vi "Rx Async.vi"(8 "error in (no error)":errorcluster, 11 "Framework in":refnum<class "Framework.lvclass">) -> (0 "error out":errorcluster, 3 "Framework out":refnum<class "Framework.lvclass">)   [LabVIEW 2017, in "DSF Core.lvlib" / "Framework.lvclass"]
uses:
  Framework.lvclass
  Framework.lvclass/Framework.ctl
  Plugin/Plugin.lvclass/Plugin.ctl
  Transfer Group/Transfer Group.lvclass/Transfer Group.ctl
  Timing/Timing.lvclass/Timing.ctl
  Buffers/Buffers.lvclass/Buffers.ctl
  Interfaces/Interface/Interface.lvclass/Interface.ctl
  Transfer Group/Increment Iteration.vi
  Transfer Group/Get Iteration.vi
  Dispatcher/Dispatch Transfer Group.vi
  Transfer Group/Get ID.vi
  Transfer Group/Copy Async to Inline.vi
  Transfer Group/Wait For Previous.vi
  Transfer Group/Update Status.vi
  Transfer Group/Get Active.vi
  Timing/Increment Iteration.vi
  Timing/Get Iteration.vi
  Interfaces/Dispatcher/Send Dispatcher Command.vi
  Buffers/Copy Async to Inline.vi
  Transfer Group/Retrieve from FIFO.vi
  Transfer Group Status/Write Status.vi
  Interfaces/Dispatcher/Write.vi
  Interfaces/Dispatcher/Write Dispatcher Command.vi
  Transfer Group/Read Return FIFO.vi
  Transfer Group/Increment Late Count.vi
  Transfer Group Status/Status Size.vi
  Interfaces/Interface/Send Command.vi
  Interfaces/Interface/Write RT FIFO.vi
  Buffer/Buffer.lvclass
  C:/Git/DSF/LabVIEW-Memory/Source/Classes/Pointer/Pointer.lvclass
  Interfaces/Dispatcher/Dispatcher Interface.lvclass
  C:/Git/DSF/Data Sharing Framework Core/Classes/Interfaces/Interface/Interface.lvclass
  Transfer Group Status/Status.lvclass
  LabVIEW-Memory/Source/Classes/Pointer/Get Address.vi
  LabVIEW-Memory/Source/Classes/Pointer/Check Size (0D).vi
  LabVIEW-Memory/Source/Classes/Pointer/Check Null Pointer.vi
  Interfaces/Interface/Errors.vi
  Interfaces/Dispatcher/Command Timeout.vi
  VIs/VI Name.vi
  Interfaces/Dispatcher/Class Name.vi
  LabVIEW-Memory/Source/Classes/Pointer/Copy All.vi
  Transfer Group/Errors.vi
  Transfer Group/Return Timeout Error.vi
  Transfer Group/Invalid Iteration Error.vi
  Plugin/Plugin.lvclass
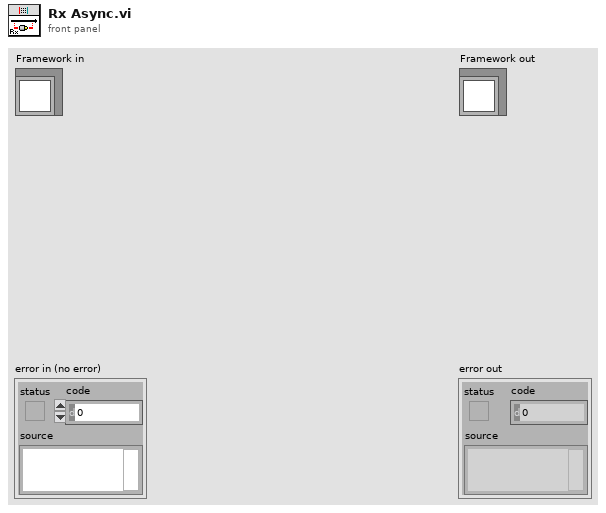
[diagram p1: front panel]
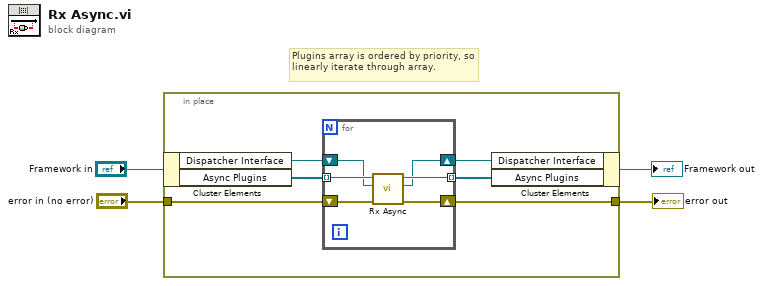
[diagram p0: block diagram]
diagram:
  # "Plugins array is ordered by priority, so linearly iterate through array."
  n1 = in-place {
    in-place-border: "error in (no error)" -> [w10]
    in-place-border: [w9] -> w3
    n2 = in-place-cluster #1("Framework in") -> ("Dispatcher Interface"=w6:refnum<class "Dispatcher Interface.lvclass">, "Async Plugins"=w8:refnum<class "Plugin.lvclass">[])
    n3 = for {
      tunnel: w8 -> [w13] mode=indexing
      tunnel: [w16] -> w7 mode=indexing
      shift-right: [w15] -> w9
      shift-left: w10 -> [w14]
      shift-right: [w11] -> w5
      shift-left: w6 -> [w12]
      n4 = call "Rx Async.vi"("error in (no error)"=w14, "Dispatcher Interface in"=w12, "Plugin in"=w13) -> ("error out"=w15:errorcluster, "Dispatcher Interface out"=w11:refnum<class "Dispatcher Interface.lvclass">, "Plugin out"=w16:refnum<class "Plugin.lvclass">)  [unwired: 6 in]
    }
    n5 = in-place-cluster #1("Dispatcher Interface"=w5, "Async Plugins"=w7) -> (→"Framework out":refnum<class "Framework.lvclass">)
  }
  "error out" <- w3
